vi "GoSlowlyToSetpoint.vi"(4 "Channel Data":T3(array[cluster]) {"Gauge Length" format="%.2f"; "Full Scale" format="%.2f"; "SI Full Scale" format="%.2f"}, 7 "Input cluster":T1 {"Set Point" format="%.2f"; "Ramp Amplitude" format="%.2f"; "Ramp Rate" format="%.2f"; "Set Point Time" format="%.2f"}, 8 "error in (no error)":errorcluster, 9 "Channels":u16[](array[ring]) items=["Channel 1", "Channel 2", "Channel 3", "Channel 4"], 10 "Axis Selector":i32[](listbox), 11 "Axis Information":T2(array[cluster])) -> (0 "Error Out":errorcluster, 1 "Channels Out":u16[](array[ring]) items=["Channel 1", "Channel 2", "Channel 3", "Channel 4"], 2 "Axis Selector Out":i32[](listbox), 3 "Axis Information Out":T2(array[cluster]))   [LabVIEW 2011]
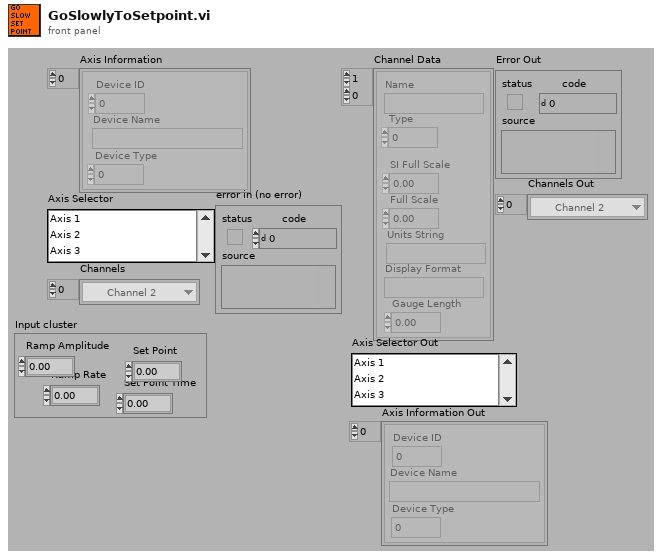
[diagram p1: front panel]
types:
  T1 = cluster{"Set Point":dbl, "Set Point Time":dbl, "Ramp Amplitude":dbl, "Ramp Rate":dbl}
  T2 = cluster{"Device ID":i32, "Device Name":string, "Device Type":i32}[]
  T3 = cluster{"Name":string, "Type":i32, "SI Full Scale":dbl, "Full Scale":dbl, "Units String":string, "Display Format":string, "Gauge Length":dbl}[][]
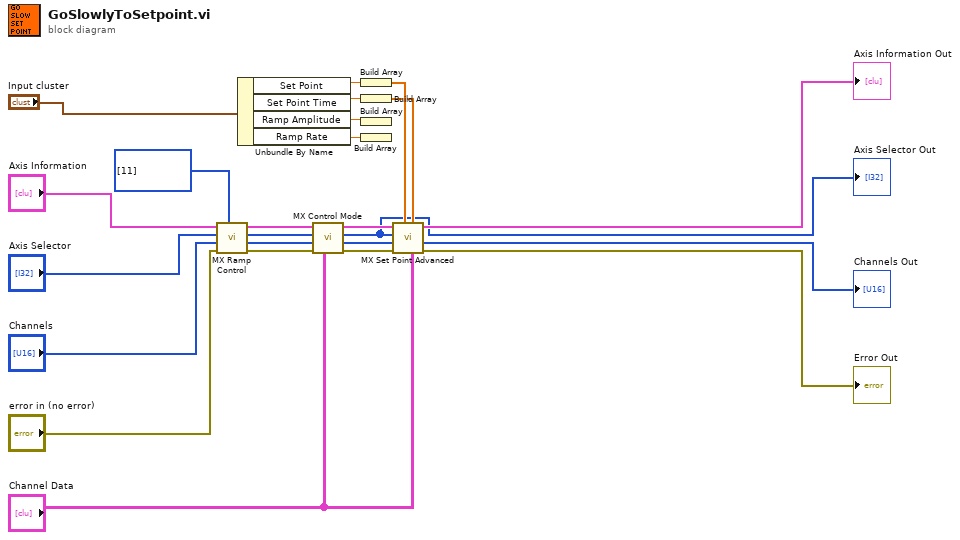
[diagram p0: block diagram]
diagram:
  w3 = u16[] [11] items=["Stop", "Start or continue", "Hold", "Continue", "Return ramp to set level at fixed rate", "Reserved", "Reserved", "Start Random without demand hold", "Start Random with demand hold", "Prepare Random Start without demand hold", "Prepare Random Start with demand hold", "Unslave", "Reserved", "Reserved", "Start Sample Data Playback or Resume", "Prepare for Start of Sample Data", "Reserved", "Reserved", "Resume Playback", "Start an electromechanical frame return"] ("Ramp Control")
  n1 = call "MX Ramp Control.vi"("Ramp Control"=w3, "error in (no error)"="error in (no error)", "Channels In"="Channels", "Axis Selector In"="Axis Selector", "Axis Information In"="Axis Information") -> ("error out"=w18:errorcluster, "Channels Out"=w19:u16[], "Axis Selector Out"=w20:i32[], "Axis Information Out"=w21:T2)  [unwired: 2 in]
  n2 = Unbundle By Name("Input cluster") -> ("Set Point"=w11:dbl, "Set Point Time"=w9:dbl, "Ramp Amplitude"=w8:dbl, "Ramp Rate"=w7:dbl)
  n3 = call "MX Control Mode.vi"("Channel Data"="Channel Data", "error in (no error)"=w18, "Control Modes"=w19, "Axis Selector"=w20, "Axis Information"=w21) -> ("error out"=w24:errorcluster, "Control Modes out"=w22:u16[], "Axis Selector out"=w2:i32[], "Axis Information out"=w23:T2)  [unwired: 1 in]
  "Axis Selector Out" <- w2
  n4 = Build Array(w11) -> (w10:dbl[])
  n5 = Build Array(w9) -> (w6:dbl[])
  n6 = Build Array(w8) -> ()  [unwired: 1 out]
  n7 = Build Array(w7) -> ()  [unwired: 1 out]
  n8 = call "MX Set Point Advanced.vi"("Channel Data"="Channel Data", "Time"=w6, "Set Point"=w10, "error in (no error)"=w24, "Channels"=w22, "Axis Selector"=w2, "Axis Information"=w23) -> ("error out"=→"Error Out":errorcluster, "Channels out"=→"Channels Out":u16[], "Axis Information out"=→"Axis Information Out":T2)  [unwired: 2 in]
